vi "PackedMatrixToFlatVector.vi"(11 "Matrix":dbl[][](array[numeric])) -> (3 "FlatVector":dbl[](array[numeric]))   [LabVIEW 2020]
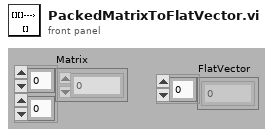
[diagram p1: front panel]
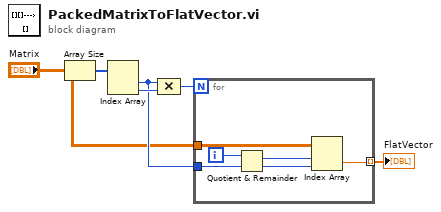
[diagram p0: block diagram]
diagram:
  n1 = Array Size(array="Matrix") -> (size(s)=w6:i32[])
  n2 = Index Array(array=w6) -> (element #1=w3:i32, element #2=w5:i32)  [unwired: 2 in]
  n3 = Compound Arithmetic op=MULTIPLY(w3, w5) -> (w4:i32)
  n4 = for {
    N: w4 -> [_]
    tunnel: w3 -> [w12]
    tunnel: [w7] -> w1 mode=indexing
    tunnel: "Matrix" -> [w10]
    i -> [w11]
    n5 = Quotient & Remainder(x=w11, y=w12) -> (x-y*floor(x/y)=w9:i32, floor(x/y)=w8:i32)
    n6 = Index Array(array=w10, index (row)=w9, index (col)=w8) -> (element=w7:dbl)
  }
  "FlatVector" <- w1
